vi "Analog Read.vi"(7 "Analog Ref Override":dbl, 8 "Error In":errorcluster, 10 "AI Channel Nums":u8[](array[numeric]), 11 "LINX Resource":T1) -> (0 "Error Out":errorcluster, 2 "Voltages":dbl[](array[numeric]), 3 "LINX Resource":T1)   [LabVIEW 2011, in "LVH-LINX.lvlib"]
uses:
  <vilib>/LabVIEW Hacker/LINX/LVH-LINX.lvlib
  Private/Type Defs/LINX Ref.ctl
  Private/Type Defs/Platform.ctl
  Private/Type Defs/Interface.ctl
  Private/Device/Type Defs/LINX Device Config.ctl
  Private/Device/Type Defs/TCP Config.ctl
  Private/Type Defs/Device Family.ctl
  Private/Type Defs/Peripheral.ctl
  <vilib>/LabVIEW Hacker/LINX/Private/Device/Device.lvlib
  <vilib>/LabVIEW Hacker/LINX/Private/myRIO/myRIO.lvlib
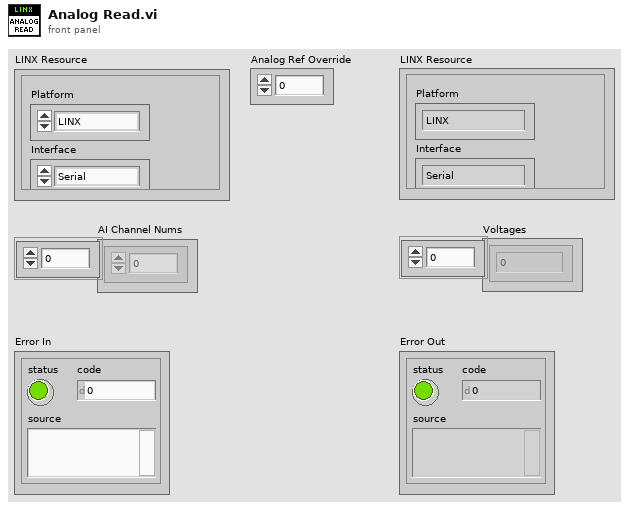
[diagram p1: front panel]
types:
  T1 = typedef "LVH-LINX.lvlib/LINX Ref.ctl" = cluster{"Platform":T2, "Interface":T3, "LINX Device Config":T4}
  T2 = typedef "LVH-LINX.lvlib/Platform.ctl" = enum16{"LINX", "myRIO"}
  T3 = typedef "LVH-LINX.lvlib/Interface.ctl" = enum16{"Serial", "TCP"}
  T4 = typedef "LVH-LINX.lvlib/Device.lvlib/LINX Device Config.ctl" = cluster{"Interface":T3, "COM Port":refnum<visa-resource-name>, "TCP Configuration":T5, "Device ID":u8, "Device Name":string, "Device Family":T6}
  T5 = typedef "LVH-LINX.lvlib/Device.lvlib/TCP Config.ctl" = cluster{"IP Address":string, "Port":dbl}
  T6 = typedef "LVH-LINX.lvlib/Device Family.ctl" = enum8{"National Instruments", "Digilent", "Arduino"}
  T7 = typedef "LVH-LINX.lvlib/Peripheral.ctl" = enum8{"DI", "DO", "AI", "AO", "PWM", "QE", "UART", "I2C", "SPI", "CAN"}
  T8 = typedef "AI.lvlib/AI Reference.ctl" = cluster{"myRIO Reference":T9, "AI Channels List":T13, "AI Scaling Constants List":T15}
  T9 = typedef "myRIO Generic Hardware Reference.ctl" = cluster{"myRIO Model":T10, "myRIO Hardware Reference":T11}
  T10 = typedef "Hardware Version Enum.ctl" = enum16{"Unknown", "myRIO-1900", "myRIO-1950"}
  T11 = typedef "myRIO v1.0 Reference.ctl" = cluster{"Generic FPGA Reference":T12, "Allow multiple opens":bool}
  T12 = typedef "Generic FPGA Reference.ctl" = refnum<k20>
  T13 = typedef "AI Channels List.ctl" = T14[]
  T14 = typedef "AI Channels Enum.ctl" = enum16{"Not Connected", "AudioIn/Left", "AudioIn/Right", "C/AI0", "C/AI1", "A/AI0", "A/AI1", "A/AI2", "A/AI3", "B/AI0", "B/AI1", "B/AI2", "B/AI3"}
  T15 = typedef "Analog Scaling Constants List.ctl" = T16[]
  T16 = typedef "Analog Scaling Constants.ctl" = cluster{"LSB Weight (Volts)":dbl, "Offset (Volts)":dbl, "Signed?":bool}
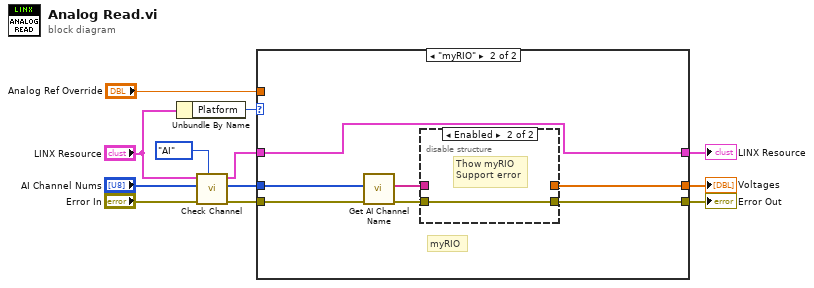
[diagram p0: block diagram]
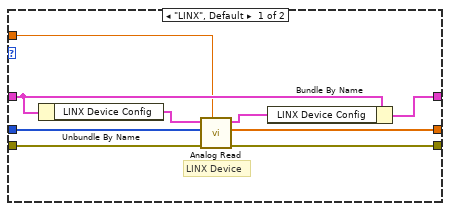
[diagram p2: hidden frame]
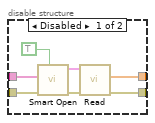
[diagram p3: hidden frame]
diagram:
  n1 = Unbundle By Name("LINX Resource") -> ("Platform"=w12:T2)
  n2 = call "Check Channel.vi"("Peripheral"=Peripheral."AI", "Error In"="Error In", "Channels"="AI Channel Nums", "LINX Resource"="LINX Resource") -> ("Error Out"=w9:errorcluster, "Channels"=w8:u8[], "LINX Resource"=w6:T1)  [unwired: 5 in]
  n3 = case shown="\"myRIO\"" w12 {
    tunnel: w9 -> [w18 w26]
    tunnel: w6 -> [w21 w28]
    tunnel: [w19 w24] -> w11
    tunnel: [w20 w28] -> w10
    tunnel: w8 -> [w15 w27]
    tunnel: [w14 w22] -> w2
    tunnel: "Analog Ref Override" -> [w13 _]
    frame "LINX", Default {
      # "LINX Device"
      n4 = Unbundle By Name(w21) -> ("LINX Device Config"=w17:T4)
      n5 = call "Analog Read.vi"("Analog Ref Override"=w13, "Error In"=w18, "AI Channels"=w15, "LINX Device Config"=w17) -> ("Error Out"=w19:errorcluster, "Voltages"=w14:dbl[], "LINX Device Config"=w16:T4)  [unwired: 5 in]
      n6 = Bundle By Name(cluster=w21, "LINX Device Config"=w16) -> (w20:T1)
    }
    frame "myRIO" {
      # "myRIO"
      n7 = call "Get AI Channel Name.vi"("Error In"=w26, "AI Channel Nums"=w27) -> ("Error Out"=w25:errorcluster, "AI Channels"=w23:string[])  [unwired: 8 in]
      n8 = disable-structure shown="Enabled" {
        disable-tunnel: w25 -> [w33 w36]
        disable-tunnel: [w32 w36] -> w24
        disable-tunnel: w23 -> [w30 _]
        disable-tunnel: [w29 _] -> w22
        frame Disabled {
          n9 = call <vilib>:"Smart Open.vi"("Allow multiple opens?"=TRUE, "error in (no error)"=w33, "Channel Names"=w30) -> ("error out"=w35:errorcluster, "AI Ref Out"=w34:T8)  [unwired: 7 in]
          n10 = call <vilib>:"Read.vi"("error in (no error)"=w35, "AI Ref In"=w34) -> ("error out"=w32:errorcluster, "Values"=w29:dbl[])  [unwired: 7 in, 1 out]
        }
        frame Enabled {
          # "Thow myRIO\nSupport error"
        }
      }
    }
  }
  "Error Out" <- w11
  "LINX Resource" <- w10
  "Voltages" <- w2
